vi "sv_Check Chirp Parameters Valid.vi"(0 "frequency range":cluster{"start (Hz)":dbl, "stop (Hz)":dbl}={"start (Hz)"=20.0, "stop (Hz)"=20000.0} {"stop (Hz)" format="%.2f"; "start (Hz)" format="%.2f"}, 1 "phase in [deg]":dbl format="%.2f", 2 "reset signal (F)":bool, 5 "chirp duration [s]":dbl=3.0, 7 "frequency spacing":enum16{"Linear", "Logarithmic"}(ring), 9 "sampling info":cluster{"Fs":dbl, "#s":u32}={"Fs"=50000.0, "#s"=50000} {"Fs" format="%.2p"}, 11 "error in (no error)":errorcluster, 12 "state in":T1={"frequency [Hz]"=20.0, "phase [rad]"=0.0, "elapsed time [s]"=0.0} {"elapsed time [s]" format="%.2f"; "phase [rad]" format="%.2f"; "frequency [Hz]" format="%.2f"}) -> (3 "t0":timestamp, 4 "frequency range out":cluster{"start (Hz)":dbl, "stop (Hz)":dbl}={"start (Hz)"=20.0, "stop (Hz)"=20000.0} {"stop (Hz)" format="%.2f"; "start (Hz)" format="%.2f"}, 6 "chirp duration [s] out":dbl, 8 "frequency spacing out":enum16{"Linear", "Logarithmic"}(ring), 10 "sampling info out":cluster{"Fs":dbl, "#s":u32}={"Fs"=50000.0, "#s"=50000} {"Fs" format="%.2p"}, 14 "state out":T1={"frequency [Hz]"=20.0, "phase [rad]"=0.0, "elapsed time [s]"=0.0} {"elapsed time [s]" format="%.2f"; "phase [rad]" format="%.2f"; "frequency [Hz]" format="%.2f"}, 15 "error out":errorcluster)   [LabVIEW 2017, in "SoundVib_Generation.lvlib"]
uses:
  <vilib>/addons/_NISVFA/_Generation/SoundVib_Generation.lvlib
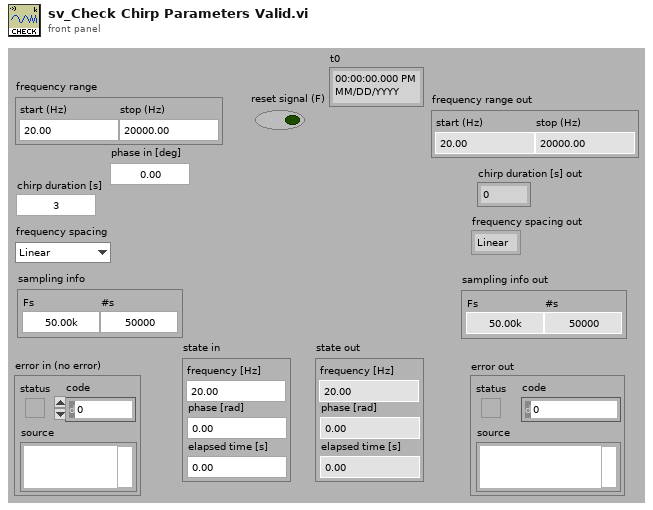
[diagram p1: front panel]
types:
  T1 = cluster{"frequency [Hz]":dbl, "phase [rad]":dbl, "elapsed time [s]":dbl}
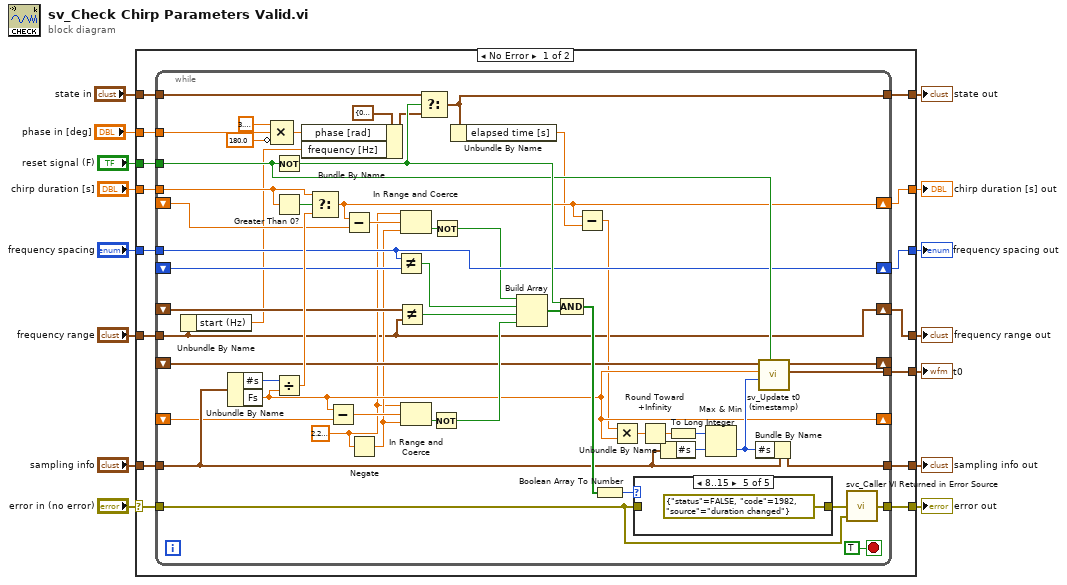
[diagram p0: block diagram]
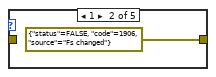
[diagram p3: hidden frame]
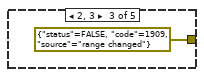
[diagram p4: hidden frame]
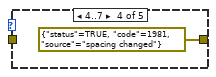
[diagram p5: hidden frame]
diagram:
  n1 = case shown="No Error" "error in (no error)" {
    selector: "error in (no error)" -> [w26 w93]
    tunnel: "frequency range" -> [w30 w90]
    tunnel: [w29 w93] -> w13
    tunnel: "frequency spacing" -> [w28 w91]
    tunnel: "chirp duration [s]" -> [w27 w92]
    tunnel: [w18 w92] -> w10
    tunnel: "reset signal (F)" -> [w24 _]
    tunnel: [w19 w91] -> w8
    tunnel: [w17 w90] -> w7
    tunnel: "sampling info" -> [w21 w89]
    tunnel: [w20 w89] -> w5
    tunnel: "phase in [deg]" -> [w25 _]
    tunnel: "state in" -> [w23 w88]
    tunnel: [w22 w88] -> w2
    tunnel: [w16 _] -> w1
    frame No Error {
      n2 = while {
        tunnel: w30 -> [w36]
        tunnel: [w82] -> w29
        tunnel: w28 -> [w54]
        tunnel: w27 -> [w75]
        tunnel: w26 -> [w73]
        tunnel: w25 -> [w33]
        tunnel: w24 -> [w55]
        tunnel: w23 -> [w69]
        tunnel: [w68] -> w22
        tunnel: w21 -> [w61]
        tunnel: [w60] -> w20
        shift-right: [w57] -> _
        shift-left: _ -> [w56]
        shift-right: [w43] -> w18
        shift-left: _ -> [w40]
        shift-right: [w54] -> w19
        shift-left: _ -> [w53]
        shift-right: [w36] -> w17
        shift-left: _ -> [w52]
        shift-right: [w51] -> _
        shift-left: _ -> [w50]
        tunnel: [w37] -> w16
        stop <- TRUE stop-if-true
        w44 = 2.220446049250313e-16
        n3 = Unbundle By Name(w36) -> ("start (Hz)"=w35:dbl)
        n4 = Unbundle By Name(w61) -> ("#s"=w71:u32, "Fs"=w51:dbl)
        n5 = Compound Arithmetic op=MULTIPLY(3.141592653589793, w33, invert 180.0 ("value")) -> (w32:dbl)
        n6 = Not(x=w55) -> (.not. x?=w64:bool)
        n7 = Greater Than 0?(x=w75) -> (x > 0?=w76:bool)
        n8 = Divide(x=w71, y=w51) -> (x/y=w74:dbl)
        n9 = Bundle By Name(cluster=T1 {"frequency [Hz]"=0.0, "phase [rad]"=0.0, "elapsed time [s]"=0.0} ("initial states"), "phase [rad]"=w32, "frequency [Hz]"=w35) -> (w63:T1)
        n10 = Select(t=w75, s=w76, f=w74) -> (s? t:f=w43:dbl)
        n11 = Subtract(x=w51, y=w50) -> (x-y=w49:dbl)
        n12 = Subtract(x=w43, y=w40) -> (x-y=w48:dbl)
        n13 = Negate(x=w44) -> (-x=w45:dbl)
        n14 = Not Equal?(x=w54, y=w53) -> (x != y?=w39:bool)
        n15 = Not Equal?(x=w52, y=w36) -> (x != y?=w81:bool)
        n16 = In Range and Coerce(upper limit=w44, x=w48, lower limit=w45) -> (In Range?=w47:bool)  [unwired: 1 out]
        n17 = In Range and Coerce(upper limit=w44, x=w49, lower limit=w45) -> (In Range?=w46:bool)  [unwired: 1 out]
        n18 = Select(t=w69, s=w64, f=w63) -> (s? t:f=w68:T1)
        n19 = Not(x=w46) -> (.not. x?=w80:bool)
        n20 = Not(x=w47) -> (.not. x?=w38:bool)
        n21 = Unbundle By Name(w68) -> ("elapsed time [s]"=w42:dbl)
        n22 = Build Array(w38, w39, w81, w80) -> (w78:bool[])
        n23 = Compound Arithmetic op=AND(w64, w78) -> (w77:bool[])
        n24 = Subtract(x=w43, y=w42) -> (x-y=w41:dbl)
        n25 = Boolean Array To Number(Boolean array=w77) -> (number=w79:u32)
        n26 = Multiply(x=w41, y=w51) -> (x*y=w66:dbl)
        n27 = case shown="8..15" w79 {
          tunnel: w73 -> [w83 _ _ _ _]
          tunnel: [w83 errorcluster {"status"=FALSE, "code"=1906, "source"="Fs changed"} ("error IO") errorcluster {"status"=FALSE, "code"=1909, "source"="range changed"} ("error IO") errorcluster {"status"=TRUE, "code"=1981, "source"="spacing changed"} ("error IO") errorcluster {"status"=FALSE, "code"=1982, "source"="duration changed"} ("error IO")] -> w72
          frame 0, Default {
          }
          frame 1 {
          }
          frame 2, 3 {
          }
          frame 4..7 {
          }
          frame 8..15 {
          }
        }
        n28 = Round Toward +Infinity(x=w66) -> (ceil(x): smallest int >= x=w67:dbl)
        n29 = Unbundle By Name(w61) -> ("#s"=w62:u32)
        n30 = To Long Integer(number=w67) -> (32bit integer=w65:i32)
        n31 = Max & Min(x=w65, y=w62) -> (min(x,y)=w59:u32)  [unwired: 1 out]
        n32 = Bundle By Name(cluster=w61, "#s"=w59) -> (w60:cluster{"Fs":dbl, "#s":u32})
        n33 = call <vilib>:"sv_Update t0 (timestamp).vi"("Reset Generation"=w55, "samples"=w59, "sample rate (S/s)"=w51, "tf previous"=w56) -> ("t0"=w37:timestamp, "tf new"=w57:timestamp)  [unwired: 5 in, 1 out]
        n34 = call <vilib>:"svc_Caller VI Returned in Error Source.vi"("warning input to caller"=w73, "error in (no error)"=w72) -> ("error out"=w82:errorcluster)  [unwired: 3 in]
      }
    }
    frame Error {
    }
  }
  "error out" <- w13
  "chirp duration [s] out" <- w10
  "frequency spacing out" <- w8
  "frequency range out" <- w7
  "sampling info out" <- w5
  "state out" <- w2
  "t0" <- w1
